vi "Create script array.vi"(0 "Modulation":cluster{"Ampl [V]":dbl, "Freq [kHz]":dbl}, 1 "Row Headers[]":string[](array[string]), 2 "Field":T2, 3 "MW Freq":T3, 4 "Orientation\nsweep [°]":dbl[](array[numeric]), 5 "Constant parameters":T4, 6 "Measurement mode":T1, 8 "Temperature\nsweep [K]":dbl[](array[numeric])) -> (7 "script array out":string[](array[string]))   [LabVIEW 2017]
uses:
  Datatypes/Constant parameters.ctl
  Datatypes/Measurement mode.ctl
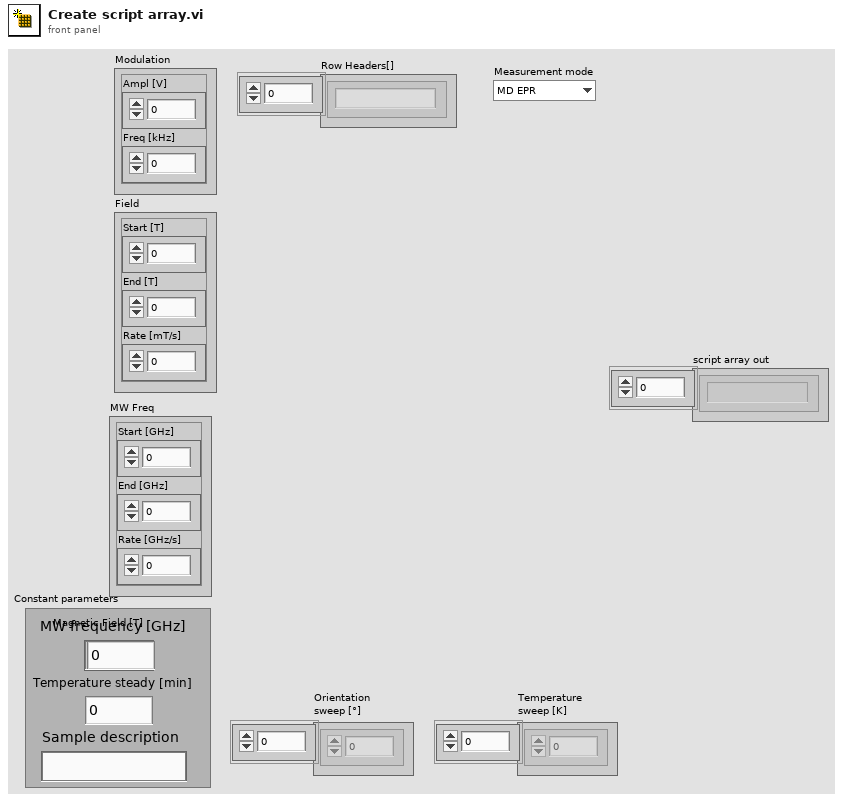
[diagram p1: front panel]
types:
  T1 = typedef "Measurement mode.ctl" = enum16{"MD EPR", "FD EPR", "EDMR", "EPR MAP"}
  T2 = cluster{"Start [T]":dbl, "End [T]":dbl, "Rate [mT/s]":dbl}
  T3 = cluster{"Start [GHz]":dbl, "End [GHz]":dbl, "Rate [GHz/s]":dbl}
  T4 = typedef "Constant parameters.ctl" = cluster{"MW frequency [GHz]":dbl, "Field [T]":dbl, "Temperature steady [min]":dbl[unit], "Sample description":string}
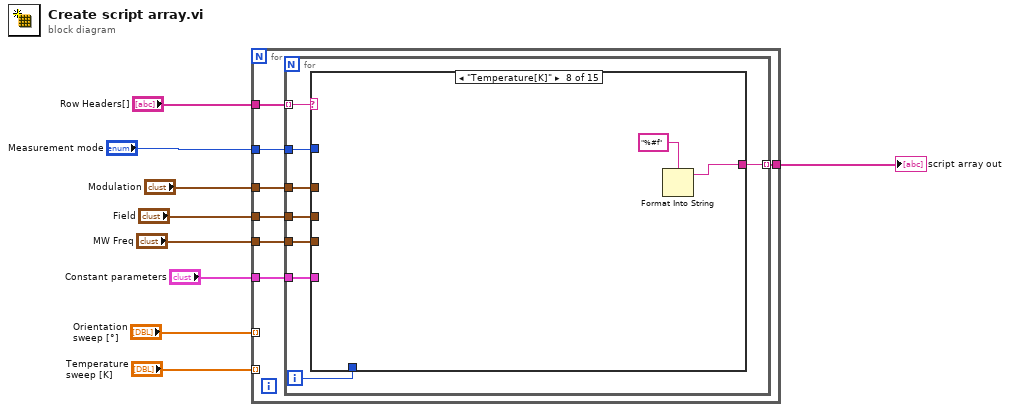
[diagram p0: block diagram]
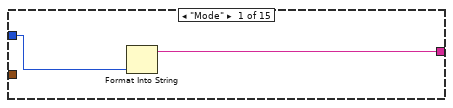
[diagram p2: hidden frame]
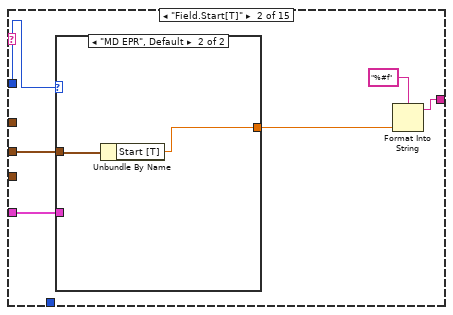
[diagram p3: hidden frame]
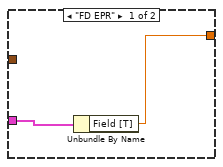
[diagram p4: hidden frame]
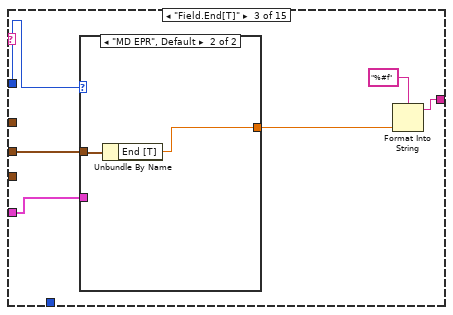
[diagram p5: hidden frame]
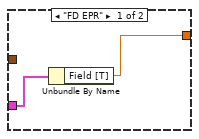
[diagram p6: hidden frame]
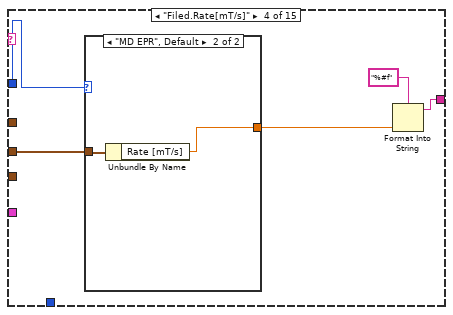
[diagram p7: hidden frame]
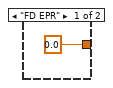
[diagram p8: hidden frame]
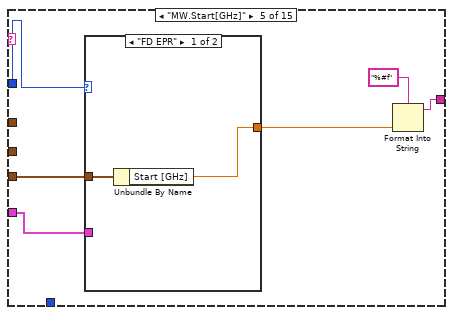
[diagram p9: hidden frame]
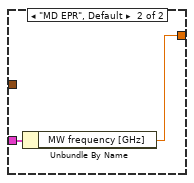
[diagram p10: hidden frame]
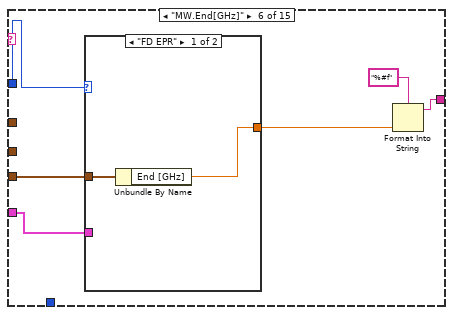
[diagram p11: hidden frame]
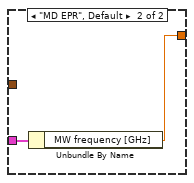
[diagram p12: hidden frame]
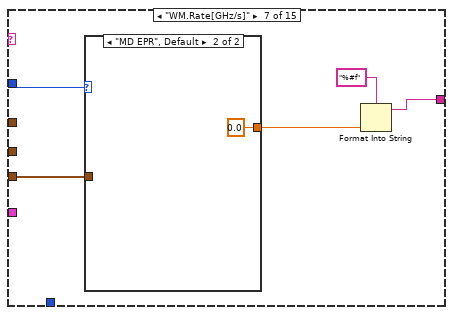
[diagram p13: hidden frame]
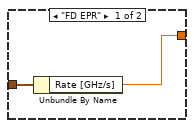
[diagram p14: hidden frame]
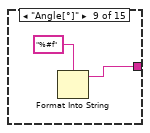
[diagram p15: hidden frame]
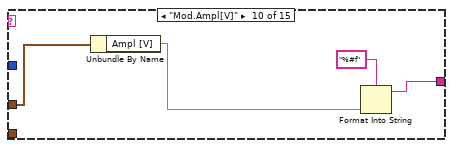
[diagram p16: hidden frame]
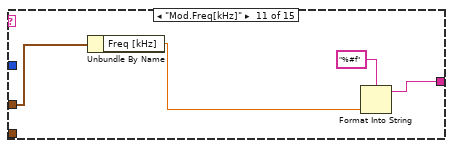
[diagram p17: hidden frame]
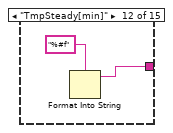
[diagram p18: hidden frame]
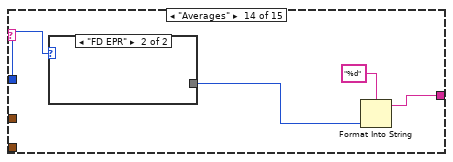
[diagram p20: hidden frame]
diagram:
  n1 = for {
    tunnel: "Measurement mode" -> [w16]
    tunnel: "Row Headers[]" -> [w15]
    tunnel: "Field" -> [w14]
    tunnel: "MW Freq" -> [w13]
    tunnel: "Modulation" -> [w12]
    tunnel: [w11] -> w6
    tunnel: "Constant parameters" -> [w10]
    tunnel: "Orientation\nsweep [°]" -> [_] mode=indexing
    tunnel: "Temperature\nsweep [K]" -> [_] mode=indexing
    n2 = for {
      tunnel: w15 -> [w24] mode=indexing
      tunnel: w16 -> [w22]
      tunnel: [w21] -> w11 mode=indexing
      tunnel: w14 -> [w20]
      tunnel: w13 -> [w19]
      tunnel: w12 -> [w18]
      tunnel: w10 -> [w17]
      i -> [w23]
      n3 = case shown="\"Temperature[K]\"" w24 {
        selector: w24 -> [_ _ _ _ _ _ _ _ _ _ _ _ _ _ w105]
        tunnel: w23 -> [_ _ _ _ _ _ _ _ _ _ _ _ _ _ _]
        tunnel: w22 -> [w26 w32 w42 w51 w60 w70 w79 _ _ _ _ _ _ w102 _]
        tunnel: [w25 w29 w39 w48 w58 w68 w77 w84 w87 w91 w95 w98 w100 w103 w105] -> w21
        tunnel: w20 -> [_ w31 w41 w50 _ _ _ _ _ _ _ _ _ _ _]
        tunnel: w19 -> [_ _ _ _ w56 w66 w75 _ _ _ _ _ _ _ _]
        tunnel: w18 -> [_ _ _ _ _ _ _ _ _ w90 w94 _ _ _ _]
        tunnel: w17 -> [_ w27 w37 _ w55 w65 _ _ _ _ _ _ _ _ _]
        frame "Mode" {
          n4 = Format Into String(w26) -> (resulting string=w25:string)  [unwired: 3 in, 1 out]
        }
        frame "Field.Start[T]" {
          n5 = case shown="\"MD EPR\", Default" w32 {
            tunnel: w31 -> [_ w36]
            tunnel: [w33 w35] -> w28
            tunnel: w27 -> [w34 _]
            frame "FD EPR" {
              n6 = Unbundle By Name(w34) -> ("Field [T]"=w33:dbl)
            }
            frame "MD EPR", Default {
              n7 = Unbundle By Name(w36) -> ("Start [T]"=w35:dbl)
            }
          }
          n8 = Format Into String(format string="%#f", w28) -> (resulting string=w29:string)  [unwired: 2 in, 1 out]
        }
        frame "Field.End[T]" {
          n9 = case shown="\"MD EPR\", Default" w42 {
            tunnel: w41 -> [_ w46]
            tunnel: w37 -> [w44 _]
            tunnel: [w43 w45] -> w38
            frame "FD EPR" {
              n10 = Unbundle By Name(w44) -> ("Field [T]"=w43:dbl)
            }
            frame "MD EPR", Default {
              n11 = Unbundle By Name(w46) -> ("End [T]"=w45:dbl)
            }
          }
          n12 = Format Into String(format string="%#f", w38) -> (resulting string=w39:string)  [unwired: 2 in, 1 out]
        }
        frame "Filed.Rate[mT/s]" {
          n13 = case shown="\"MD EPR\", Default" w51 {
            tunnel: w50 -> [_ w54]
            tunnel: [0.0 w53] -> w47
            frame "FD EPR" {
            }
            frame "MD EPR", Default {
              n14 = Unbundle By Name(w54) -> ("Rate [mT/s]"=w53:dbl)
            }
          }
          n15 = Format Into String(format string="%#f", w47) -> (resulting string=w48:string)  [unwired: 2 in, 1 out]
        }
        frame "MW.Start[GHz]" {
          n16 = case shown="\"FD EPR\"" w60 {
            tunnel: [w61 w63] -> w57
            tunnel: w56 -> [w62 _]
            tunnel: w55 -> [_ w64]
            frame "FD EPR" {
              n17 = Unbundle By Name(w62) -> ("Start [GHz]"=w61:dbl)
            }
            frame "MD EPR", Default {
              n18 = Unbundle By Name(w64) -> ("MW frequency [GHz]"=w63:dbl)
            }
          }
          n19 = Format Into String(format string="%#f", w57) -> (resulting string=w58:string)  [unwired: 2 in, 1 out]
        }
        frame "MW.End[GHz]" {
          n20 = case shown="\"FD EPR\"" w70 {
            tunnel: [w71 w73] -> w67
            tunnel: w66 -> [w72 _]
            tunnel: w65 -> [_ w74]
            frame "FD EPR" {
              n21 = Unbundle By Name(w72) -> ("End [GHz]"=w71:dbl)
            }
            frame "MD EPR", Default {
              n22 = Unbundle By Name(w74) -> ("MW frequency [GHz]"=w73:dbl)
            }
          }
          n23 = Format Into String(format string="%#f", w67) -> (resulting string=w68:string)  [unwired: 2 in, 1 out]
        }
        frame "WM.Rate[GHz/s]" {
          n24 = case shown="\"MD EPR\", Default" w79 {
            tunnel: [w80 0.0 ("Rate [GHz/s]")] -> w76
            tunnel: w75 -> [w81 _]
            frame "FD EPR" {
              n25 = Unbundle By Name(w81) -> ("Rate [GHz/s]"=w80:dbl)
            }
            frame "MD EPR", Default {
            }
          }
          n26 = Format Into String(format string="%#f", w76) -> (resulting string=w77:string)  [unwired: 2 in, 1 out]
        }
        frame "Temperature[K]" {
          n27 = Format Into String(format string="%#f") -> (resulting string=w84:string, w83:dbl)  [unwired: 2 in, 1 out]
        }
        frame "Angle[°]" {
          n28 = Format Into String(format string="%#f") -> (resulting string=w87:string, w86:dbl)  [unwired: 2 in, 1 out]
        }
        frame "Mod.Ampl[V]" {
          n29 = Unbundle By Name(w90) -> ("Ampl [V]"=w89:dbl)
          n30 = Format Into String(format string="%#f", w89) -> (resulting string=w91:string)  [unwired: 2 in, 1 out]
        }
        frame "Mod.Freq[kHz]" {
          n31 = Unbundle By Name(w94) -> ("Freq [kHz]"=w93:dbl)
          n32 = Format Into String(format string="%#f", w93) -> (resulting string=w95:string)  [unwired: 2 in, 1 out]
        }
        frame "TmpSteady[min]" {
          n33 = Format Into String(format string="%#f") -> (resulting string=w98:string, w97:dbl[unit])  [unwired: 2 in, 1 out]
        }
        frame "Description" {
        }
        frame "Averages" {
          n34 = Format Into String(format string="%d") -> (resulting string=w103:string, w101:i64)  [unwired: 2 in, 1 out]
          n35 = case shown="\"FD EPR\"" w102 {
            tunnel: w101 -> [_ _]
            frame "MD EPR", Default {
            }
            frame "FD EPR" {
            }
          }
        }
        frame "Ignored", Default {
        }
      }
    }
  }
  "script array out" <- w6
